vi "Prime Pump Impl.vi"(6 "Cycles":u16=5, 8 "error in (no error)":errorcluster, 9 "Waste Valve Pos.":u16=2, 10 "Buffer Val Pos.":u16=3, 11 "Alltesta Autosampler in":refnum<class "Alltesta Autosampler.lvclass">) -> (0 "error out":errorcluster, 3 "Alltesta Autosampler out":refnum<class "Alltesta Autosampler.lvclass">)   [LabVIEW 2023, in "Alltesta Autosampler.lvlib" / "Alltesta Autosampler.lvclass"]
uses:
  Alltesta Autosampler.lvclass
  Alltesta Autosampler.lvclass/Alltesta Autosampler.ctl
  Autosampler/Autosampler.lvclass
  C:/FLASH/Development/Hardware/Autosampler/Autosampler.lvclass
  C:/FLASH/Development/Hardware/Device/Device.lvclass
  C:/Program Files/National Instruments/LabVIEW 2023/vi.lib/ActorFramework/Actor/Actor.lvclass
  C:/FLASH/Development/Hardware/Alltesta Autosampler/Alltesta Autosampler.lvclass
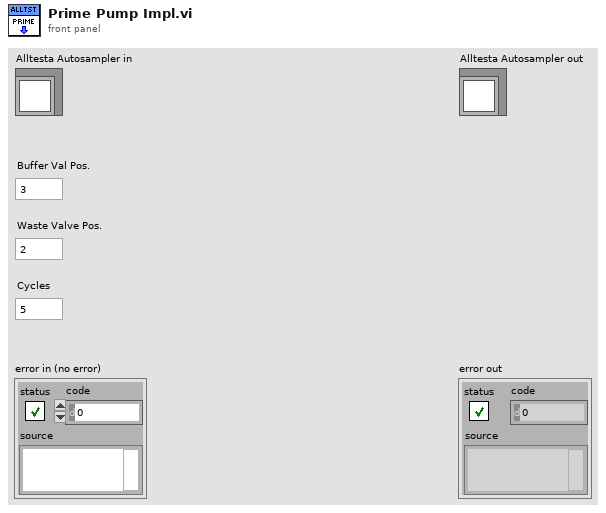
[diagram p1: front panel]
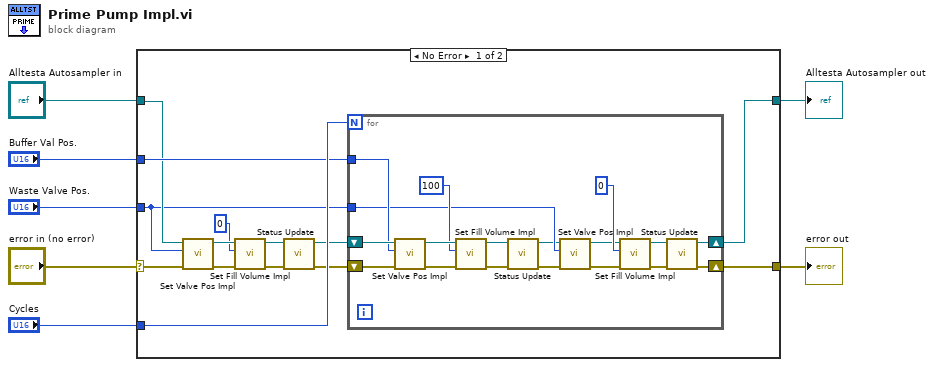
[diagram p0: block diagram]
diagram:
  n1 = case shown="No Error" "error in (no error)" {
    selector: "error in (no error)" -> [w17 w41]
    tunnel: [w20 w41] -> w6
    tunnel: "Alltesta Autosampler in" -> [w16 w40]
    tunnel: [w19 w40] -> w4
    tunnel: "Cycles" -> [w21 _]
    tunnel: "Waste Valve Pos." -> [w12 _]
    tunnel: "Buffer Val Pos." -> [w18 _]
    frame No Error {
      n2 = call-dynamic "Set Valve Pos Impl.vi"("error in (no error)"=w17, "Valve Pos"=w12, "Alltesta Autosampler in"=w16) -> ("error out"=w14:errorcluster, "Alltesta Autosampler out"=w15:refnum<class "Alltesta Autosampler.lvclass">)  [unwired: 7 in]
      n3 = call-dynamic "Set Fill Volume Impl.vi"("error in (no error)"=w14, "Volume, uL"=u16 0, "Alltesta Autosampler in"=w15) -> ("error out"=w11:errorcluster, "Alltesta Autosampler out"=w10:refnum<class "Alltesta Autosampler.lvclass">)  [unwired: 7 in]
      n4 = call "Status Update.vi"("error in (no error)"=w11, "Autosampler in"=w10) -> ("error out"=w8:errorcluster, "Autosampler out"=w9:refnum<class "Alltesta Autosampler.lvclass">)  [unwired: 7 in, 1 out]
      n5 = for {
        N: w21 -> [_]
        shift-right: [w22] -> w20
        shift-left: w8 -> [w39]
        shift-right: [w23] -> w19
        shift-left: w9 -> [w38]
        tunnel: w18 -> [w35]
        tunnel: w12 -> [w33]
        n6 = call-dynamic "Set Valve Pos Impl.vi"("error in (no error)"=w39, "Valve Pos"=w35, "Alltesta Autosampler in"=w38) -> ("error out"=w37:errorcluster, "Alltesta Autosampler out"=w36:refnum<class "Alltesta Autosampler.lvclass">)  [unwired: 7 in]
        n7 = call-dynamic "Set Fill Volume Impl.vi"("error in (no error)"=w37, "Volume, uL"=u16 100, "Alltesta Autosampler in"=w36) -> ("error out"=w29:errorcluster, "Alltesta Autosampler out"=w28:refnum<class "Alltesta Autosampler.lvclass">)  [unwired: 7 in]
        n8 = call "Status Update.vi"("error in (no error)"=w29, "Autosampler in"=w28) -> ("error out"=w26:errorcluster, "Autosampler out"=w27:refnum<class "Alltesta Autosampler.lvclass">)  [unwired: 7 in, 1 out]
        n9 = call-dynamic "Set Valve Pos Impl.vi"("error in (no error)"=w26, "Valve Pos"=w33, "Alltesta Autosampler in"=w27) -> ("error out"=w30:errorcluster, "Alltesta Autosampler out"=w31:refnum<class "Alltesta Autosampler.lvclass">)  [unwired: 7 in]
        n10 = call-dynamic "Set Fill Volume Impl.vi"("error in (no error)"=w30, "Volume, uL"=u16 0, "Alltesta Autosampler in"=w31) -> ("error out"=w25:errorcluster, "Alltesta Autosampler out"=w24:refnum<class "Alltesta Autosampler.lvclass">)  [unwired: 7 in]
        n11 = call "Status Update.vi"("error in (no error)"=w25, "Autosampler in"=w24) -> ("error out"=w22:errorcluster, "Autosampler out"=w23:refnum<class "Alltesta Autosampler.lvclass">)  [unwired: 7 in, 1 out]
      }
    }
    frame Error {
    }
  }
  "error out" <- w6
  "Alltesta Autosampler out" <- w4
